vi "solenoid_single_okta.vi"(10 "INPUT_OKTA":bool, 11 "INPUT":bool) -> (3 "OUTPUT_POSITIVE":bool)   [LabVIEW 2013]
panel:
  # "Single Coil Solenoid with OK TO Actuate\n\nInput is the desired state of the solenoid\nOKTA is the ok to actuate state for the solenoid\nIf OKTA is not set thn the solenoid is not set\nThis replicates the SW interface of the dual coil solenoid block but provides no safety, as the output could actuate when OKTA is cleared."
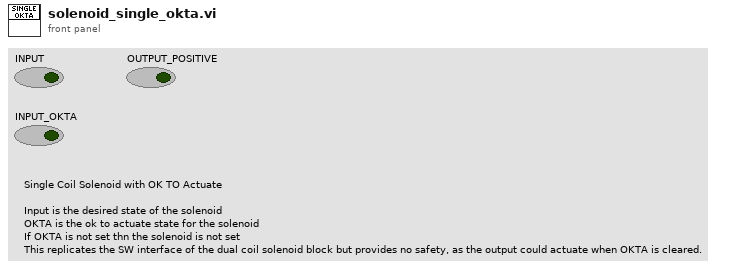
[diagram p1: front panel]
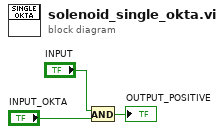
[diagram p0: block diagram]
diagram:
  n1 = And(x="INPUT", y="INPUT_OKTA") -> (x .and. y?=→"OUTPUT_POSITIVE":bool)
